vi "T3.vi"() -> ()   [LabVIEW 2020]
panel:
  out "Valoare absoluta":dbl
  in  "A":dbl
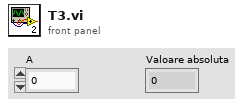
[diagram p1: front panel]
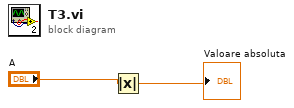
[diagram p0: block diagram]
diagram:
  n1 = Absolute Value(x="A") -> (abs(x)=→"Valoare absoluta":dbl)
